vi "AprilTag Target Package Code 2.vi"() -> ()   [LabVIEW 2025]
uses:
  Camera Info.ctl
  <vilib>/vision/Shape Detection.llb/ShapeDetectionMatchOptions.ctl
  <vilib>/vision/Pattern Matching.llb/IMAQ Match Range Setting.ctl
  <vilib>/vision/Pattern Matching.llb/IMAQ Curve Parameters.ctl
  State Machine/AprialTag Main Cluster.ctl
  State Machine/AprialTag States.ctl
  <vilib>/vision/Image Controls.llb/IMAQ Image.ctl
  Steam Type.ctl
  Camera Set Up/Event/Event Setup Types.ctl
  <vilib>/Utility/config.llb/Read Key (String).vi
  <vilib>/Utility/config.llb/Write Key (String).vi
  <vilib>/Utility/config.llb/NI_LVConfig.lvlib
  <vilib>/vision/NI_Vision_Development_Module.lvlib
  <vilib>/ptbypt/NI_PtbyPt.lvlib
panel:
  in  "Main":enum32{"Page 1", "Page 2"}(tab)
  out "Target Pitch":dbl[](array[numeric]) caption="Tag Pitch (deg)" format="%.1f"
  out "Target Yaw":dbl[](array[numeric]) caption="Tag Yaw (deg)" format="%.1f"
  out "Tag ID":i32[](array[numeric]) caption="Tag Number"
  out "Image":T1(plugin-control)
  in  "Camera Name":string="cam0"
  in  "Settings":bool
  in  "Save":bool
  in  "Tools":bool
  out "FPS":dbl format="%#.0f"
  out "Distance":dbl[](array[numeric]) caption="Tag Distance (in)" format="%.1f"
  out "Angle":dbl[](array[numeric]) caption="Center Angle (deg)" format="%.1f"
  out "Height":u32=360
  out "Width":u32=640
  out "Waveform Chart":dbl[](graph)
  out "Treshold":T1(plugin-control)
  in  "Curve Parameters":T2={"Extraction Mode"=0, "Edge Threshold"=100, "Edge Filter Size"=1, "Min Length"=10, "Row Search Step Size"=75, "Col Search Step Size"=75, "Max Endpoint Gap"=10, "Closed"=TRUE, "Subpixel"=FALSE} {"Max Endpoint Gap" min=0; "Col Search Step Size" min=1 max=255 step=1; "Row Search Step Size" min=1 max=255 step=1; "Min Length" min=0; "Edge Filter Size" items=["Fine", "Normal", "Controur Tracing"]; "Edge Threshold" min=1 max=65535 step=1; "Extraction Mode" items=["Normal", "Uniform Regions"]}
  in  "Minimum match score":dbl=100.0
  in  "Home":bool
  in  "Robot Calibration Cluster":T3={"Camera Height on robot (in)"=9.5, "Camera Angle on the robot (deg)"=2.5, "Camera FOV Vert View Angle (deg)"=26.5, "Camera FOV Hor View Angle (deg)"=68.5, "Camera Focal Length (mm)"=10.0, "Target size (in)"=6.5} {"Camera FOV Hor View Angle (deg)" format="%#_13g"; "Camera Focal Length (mm)" format="%#_13g"; "Target size (in)" format="%#_13g"; "Camera FOV Vert View Angle (deg)" format="%#_13g"; "Camera Angle on the robot (deg)" format="%#_13g"; "Camera Height on robot (in)" format="%#_13g"}
  in  "Max Rect Size (pix)":dbl=12000.0
  in  "Min Rect Size (pix)":dbl=50.0
  in  "Match Options":T4={"Rotation"=TRUE, "Scale"=TRUE, "Occlusion"=FALSE, "Range Settings"=[{"Match Constraints"=0, "Min"=-25.0, "Max"=25.0}, {"Match Constraints"=1, "Min"=25.0, "Max"=200.0}]} {"Range Settings"."Match Constraints" items=["Rotation Angle (degrees)", "Scale Factor (%)", "Occlusion (%)"]}
  in  "Range":cluster{"Lower value":sgl, "Upper value":sgl}={"Lower value"=128.0, "Upper value"=255.0} {"Upper value" format="%.2f"; "Lower value" format="%.2f"}
  # "Edit the camera name to the camera that you are going to use for this target package"
  # "Range"
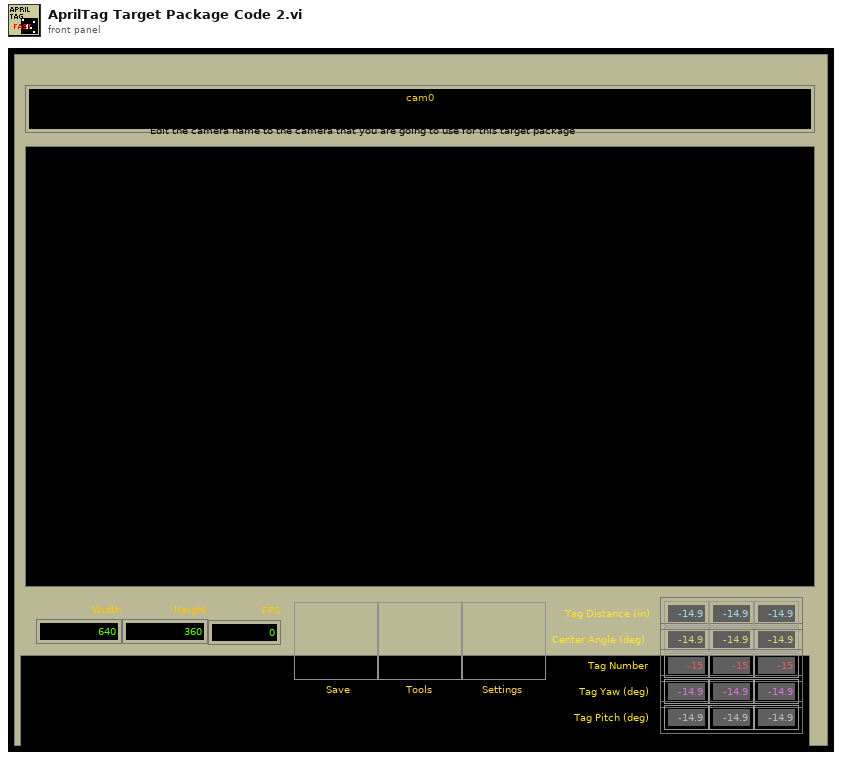
[diagram p1: front panel]
types:
  T1 = typedef "IMAQ Image.ctl" = refnum<image>
  T2 = typedef "IMAQ Curve Parameters.ctl" = cluster{"Extraction Mode":u32, "Edge Threshold":i32, "Edge Filter Size":u32, "Min Length":i32, "Row Search Step Size":i32, "Col Search Step Size":i32, "Max Endpoint Gap":i32, "Closed":bool, "Subpixel":bool}
  T3 = typedef "Camera Info.ctl" = cluster{"Camera Height on robot (in)":dbl, "Camera Angle on the robot (deg)":dbl, "Camera FOV Vert View Angle (deg)":dbl, "Camera FOV Hor View Angle (deg)":dbl, "Camera Focal Length (mm)":dbl, "Target size (in)":dbl}
  T4 = typedef "ShapeDetectionMatchOptions.ctl" = cluster{"Rotation":bool, "Scale":bool, "Occlusion":bool, "Range Settings":T5[]}
  T5 = typedef "IMAQ Match Range Setting.ctl" = cluster{"Match Constraints":u32, "Min":dbl, "Max":dbl}
  T6 = typedef "AprialTag States.ctl" = enum16{"Message Dispatcher", "INI", "Open", "Save", "Exit"}
  T7 = typedef "AprialTag Main Cluster.ctl" = cluster{"AprilTage FIFO":T6[], "Camera Name":string, "AprilTag path":path, "Control Ref's":refnum<vi>[], "Main Image":T1, "EDIT Settings":bool, "Calibration path":path, "Camera Number":dbl}
  T8 = cluster{"Min Width":dbl, "Max Width":dbl, "Min Height":dbl, "Max Height":dbl}
  T9 = typedef "Steam Type.ctl" = enum8{"Unknown", "Apriltag", "Fuel", "Other"}
  T10 = typedef "Event Setup Types.ctl" = enum16{"Default", "Camera Loop Started", "GreyScale", "Reset Team Number", "Save Data", "Exit"}
  T11 = typedef "Image Type" = u32
  T12 = cluster{"Corners":cluster{"X":sgl, "Y":sgl}[], "Angle":dbl, "Width":dbl, "Height":dbl, "Score":dbl}[]
  T13 = typedef "AprilTag Target Fields.ctl" = cluster{"diameter points":cluster{"first point":cluster{"x":dbl, "y":dbl}, "projected point":cluster{"x":dbl, "y":dbl}}, "normalized center":cluster{"x":dbl, "y":dbl}, "Overall Score":dbl, "Distance (ft)":dbl, "Offset Angle":dbl, "Tag corner points":cluster{"X":dbl, "Y":dbl}[], "Tag Center":cluster{"X":dbl, "Y":dbl}, "Tag Yaw":dbl, "Tag Pitch":dbl, "Target Roll (deg)":dbl, "AprilTag Number":i32, "homography matrix":dbl[]}
  T14 = typedef "NI_LVConfig.lvlib/Config Data RefNum.ctl" = refnum<k1>
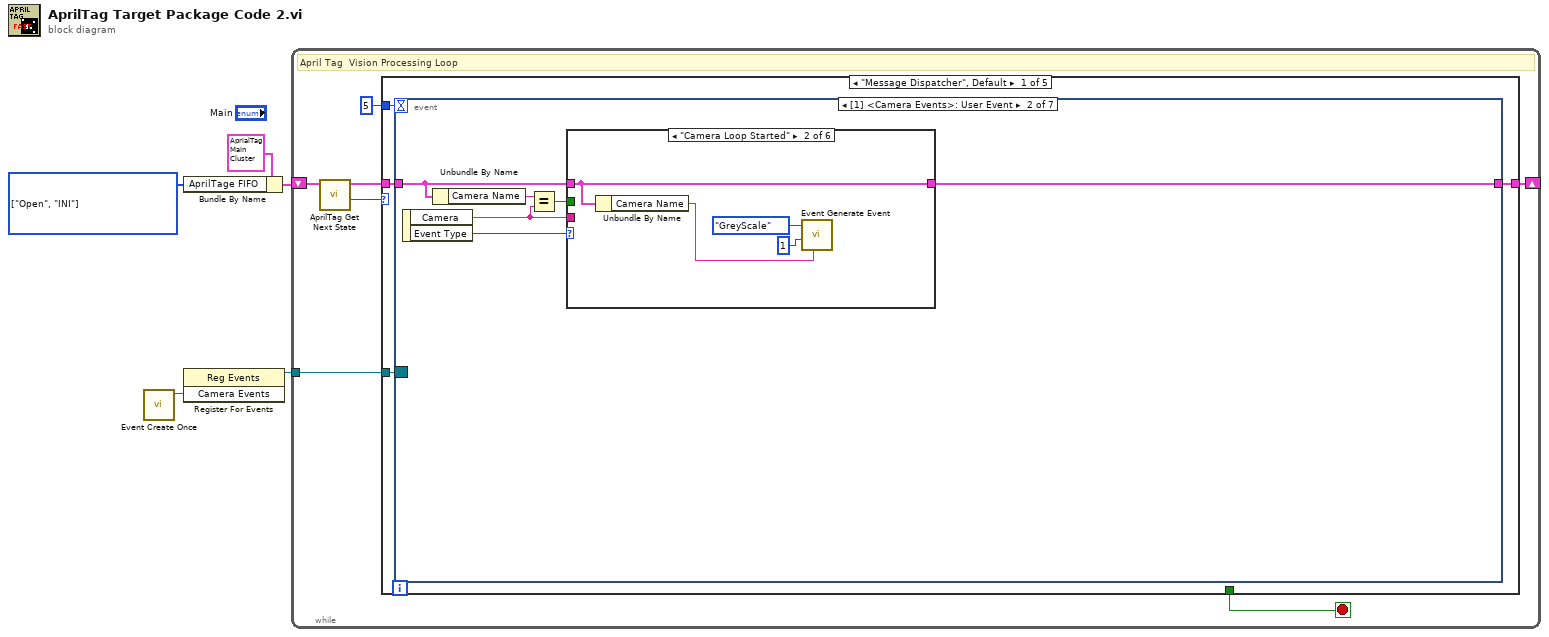
[diagram p0: block diagram]
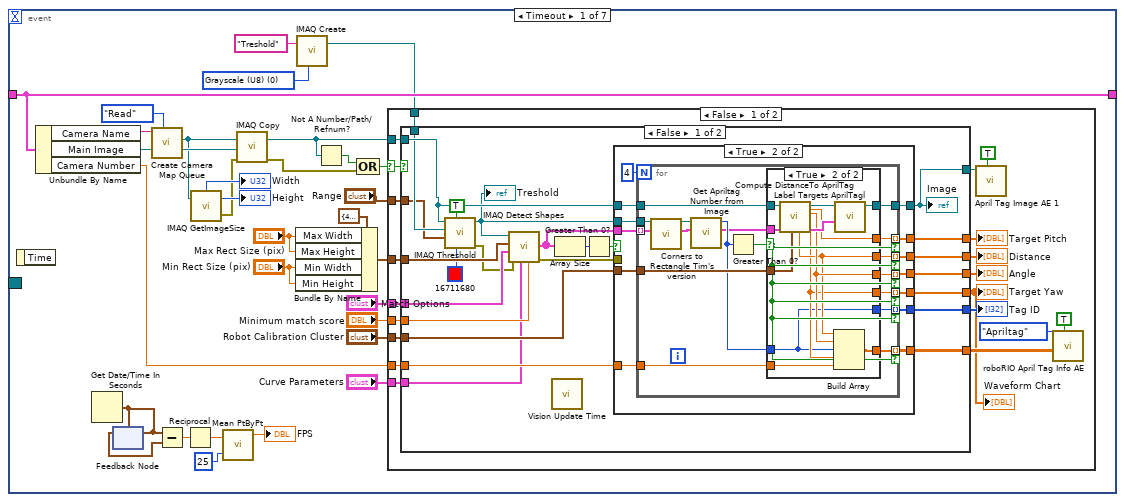
[diagram p2: hidden frame]
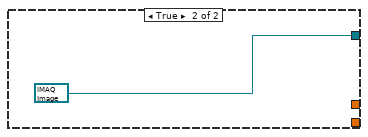
[diagram p5: hidden frame]
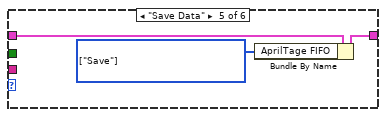
[diagram p10: hidden frame]
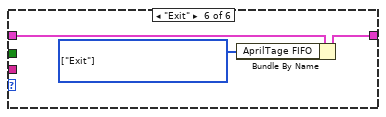
[diagram p11: hidden frame]
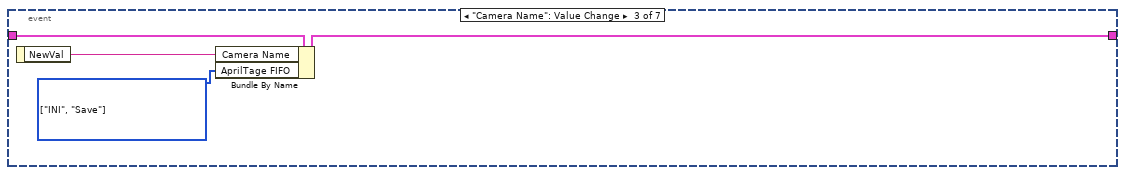
[diagram p12: hidden frame]
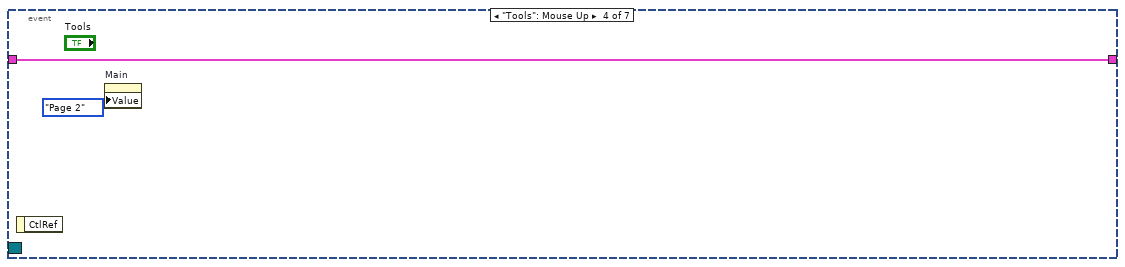
[diagram p13: hidden frame]
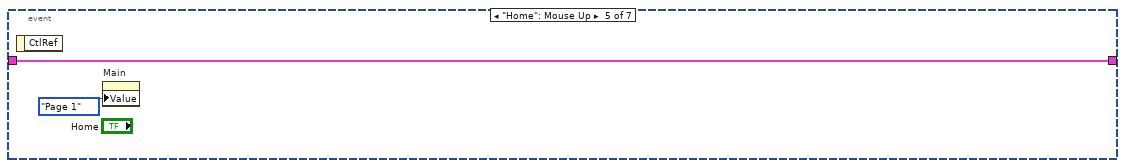
[diagram p14: hidden frame]
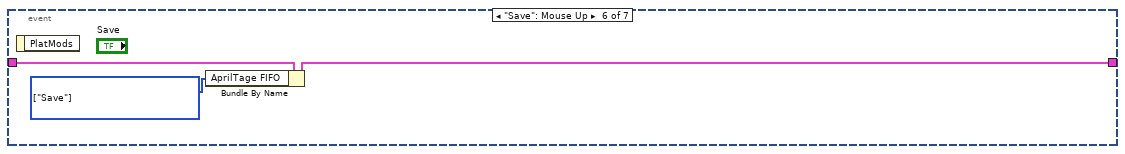
[diagram p15: hidden frame]
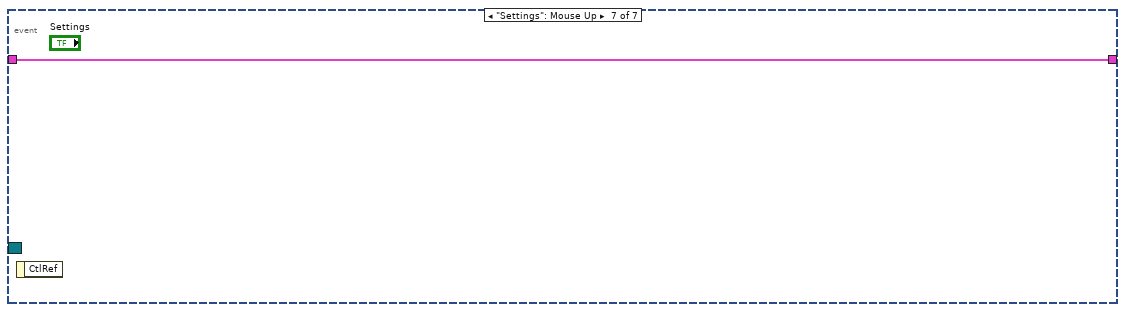
[diagram p16: hidden frame]
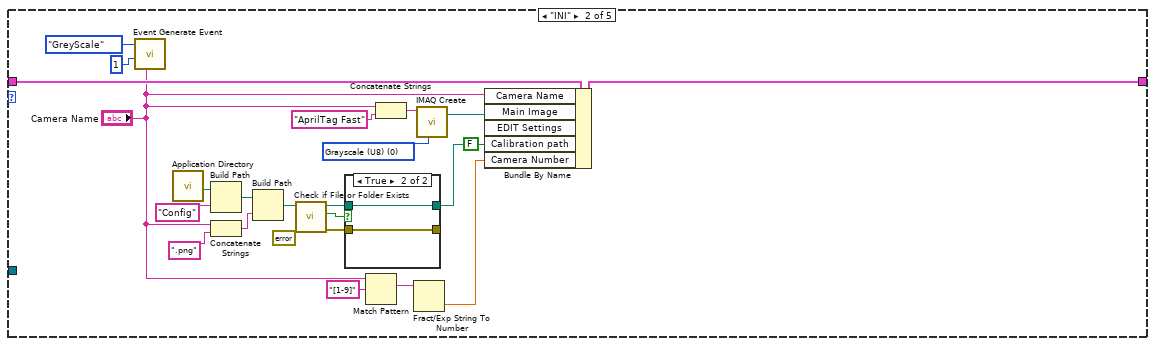
[diagram p17: hidden frame]
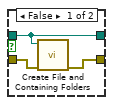
[diagram p18: hidden frame]
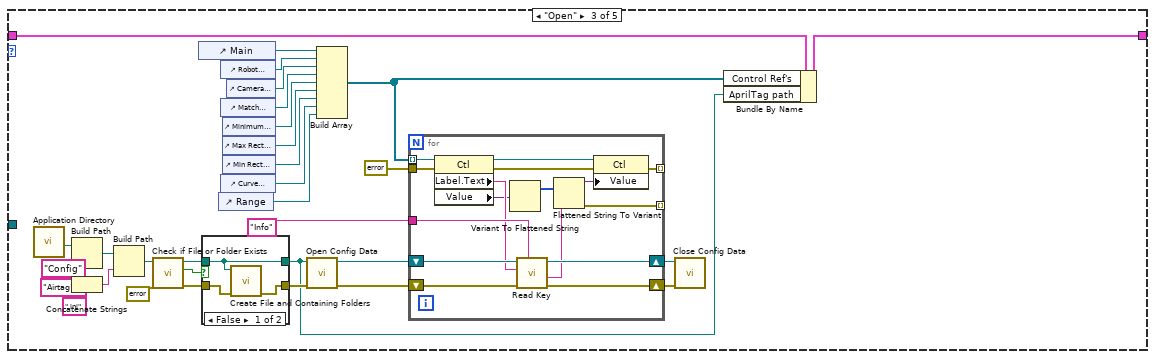
[diagram p19: hidden frame]
diagram:
  w1 = T6[] [enum."Open", enum."INI"] items=["Message Dispatcher", "INI", "Open", "Save", "Exit"] ("AprilTage FIFO")
  n1 = call "Event Create Once.vi"() -> ("Camera Events"=w5:refnum<user-event>)  [unwired: 10 in, 1 out]
  n2 = Bundle By Name(cluster=T7 {"AprilTage FIFO"=[], "Camera Name"="", "AprilTag path"=path "", "Control Ref's"=[], "Main Image"=refnum, "EDIT Settings"=FALSE, "Calibration path"=path "", "Camera Number"=0.0} ("AprilTag Main Cluster out"), "AprilTage FIFO"=w1) -> (w2:T7)
  n3 = register-events(w5) -> (reference out=w4:refnum<event-registration>)  [unwired: 2 in, 1 out]
  n4 = while {
    tunnel: w4 -> [w12]
    shift-right: [w8] -> _
    shift-left: w2 -> [w7]
    stop <- w11 stop-if-true
    # "April Tag  Vision Processing Loop"
    n5 = call "AprilTag Get Next State.vi"("AprilTag Main Cluster in"=w7) -> ("Next State"=w9:T6, "AprilTag Main Cluster out"=w10:T7)  [unwired: 9 in]
    n6 = case shown="\"Message Dispatcher\", Default" w9 {
      tunnel: w12 -> [w16 _ _ _ _]
      tunnel: [_ _ _ _ TRUE] -> w11
      tunnel: w10 -> [w14 w191 w214 w252 w268]
      tunnel: [w15 w190 w212 w252 w268] -> w8
      tunnel: 5 ("Timeout") -> [w13 _ _ _ _]
      frame "Message Dispatcher", Default {
        n7 = event shown="[1] <Camera Events>: User Event" {
          selector: w16 -> [_ _ _ _ _ _ _]
          dyn-events: _ -> [_ _ _ _ _ _ _]
          timeout: w13 -> [_ _ _ _ _ _ _]
          tunnel: w14 -> [w47 w140 w159 w160 w162 w166 w167]
          tunnel: [w47 w142 w158 w160 w162 w165 w167] -> w15
          event Timeout {
            w20 = T11 0 items=["Grayscale (U8)", "Grayscale (I16)", "Grayscale (SGL)", "Complex (CSG)", "RGB (U32)", "HSL (U32)", "RGB (U64)", "Grayscale (U16)"] ("Image Type")
            n8 = event-data() -> ()  [unwired: 1 in, 1 out]
            n9 = Unbundle By Name(w47) -> ("Camera Name"=w45:string, "Main Image"=w27:T1, "Camera Number"=w44:dbl)
            n10 = Get Date/Time In Seconds() -> (seconds since 1Jan1904=w33:timestamp)
            n11 = feedback-in #1(w33) -> ()
            n12 = feedback #1(w33) -> (w34:timestamp)
            n13 = call "Create Camera Map Queue.vi"("Action"=enum16{"Read", "Write"}."Read", "Camera"=w45) -> ("Image out"=w24:T1)  [unwired: 8 in, 1 out]
            n14 = Subtract(x=w33, y=w34) -> (x-y=w32:dbl)
            n15 = Reciprocal(x=w32) -> (1/x=w31:dbl)
            n16 = call "IMAQ GetImageSize"("Image"=w24) -> ("Y Resolution"=→"Height":i32, "X Resolution"=→"Width":i32, "error out"=w21:errorcluster)  [unwired: 3 in]
            n17 = call <vilib>:"Mean PtByPt.vi"("x"=w31, "sample length"=25) -> ("mean"=→"FPS":dbl)  [unwired: 2 in, 1 out]
            n18 = call "IMAQ Copy"("error in (no error)"=w21, "Image Dst"=w27, "Image Src"=w24) -> ("error out"=w25:errorcluster, "Image Dst Out"=w26:T1)  [unwired: 3 in]
            n19 = Bundle By Name(cluster=T8 {"Min Width"=40.0, "Max Width"=100.0, "Min Height"=40.0, "Max Height"=200.0} ("Rectangle Descriptor"), "Max Width"="Max Rect Size (pix)", "Max Height"="Max Rect Size (pix)", "Min Width"="Min Rect Size (pix)", "Min Height"="Min Rect Size (pix)") -> (w43:T8)
            n20 = call "IMAQ Create"("Image Name"="Treshold", "Image Type"=w20) -> ("New Image"=w18:T1)  [unwired: 2 in, 2 out]
            n21 = Not A Number/Path/Refnum?(number/path/refnum=w26) -> (NaN/Path/Refnum?=w36:bool)
            n22 = Compound Arithmetic op=OR(w36, w25) -> (w35:bool)
            n23 = case shown="False" w35 {
              selector: w35 -> [w51 _]
              tunnel: "Robot Calibration Cluster" -> [w66 _]
              tunnel: w26 -> [w61 _]
              tunnel: w44 -> [w60 _]
              tunnel: w43 -> [w58 _]
              tunnel: "Match Options" -> [w57 _]
              tunnel: "Minimum match score" -> [w56 _]
              tunnel: "Curve Parameters" -> [w52 _]
              tunnel: w18 -> [w50 _]
              tunnel: "Range" -> [w49 _]
              frame False {
                n24 = case shown="False" w51 {
                  tunnel: w66 -> [w91 _]
                  tunnel: [w89 _] -> w67
                  tunnel: [w88 _] -> w65
                  tunnel: [w87 _] -> w48
                  tunnel: [w86 _] -> w64
                  tunnel: [w85 _] -> w63
                  tunnel: [w84 _] -> w62
                  tunnel: w61 -> [w74 _]
                  tunnel: w60 -> [w83 _]
                  tunnel: [w82 T1 refnum ("Image out")] -> w59
                  tunnel: w58 -> [w81 _]
                  tunnel: w57 -> [w78 _]
                  tunnel: w56 -> [w77 _]
                  tunnel: w52 -> [w75 _]
                  tunnel: w50 -> [w72 _]
                  tunnel: w49 -> [w71 _]
                  frame False {
                    n25 = call "IMAQ Threshold"("Replace Value"=u32 16711680, "Keep/Replace Value (Replace)"=TRUE, "Range"=w71, "Image Dst"=w72, "Image Src"=w74) -> ("error out"=w69:errorcluster, "Image Dst Out"=w68:T1)  [unwired: 5 in]
                    "Treshold" <- w68
                    n26 = call-poly "IMAQ Detect Shapes"("Minimum match score"=w77, "Curve Parameters"=w75, "error in (no error)"=w69, "Match Options"=w78, "Rectangle Descriptor"=w81, "Image"=w68) -> ("error out"=w79:errorcluster, "Rectangles"=w80:T12)  [unwired: 3 in, 1 out]
                    n27 = call "Vision Update Time.vi"() -> ()  [unwired: 12 in]
                    n28 = Array Size(array=w80) -> (size(s)=w76:i32)
                    n29 = Greater Than 0?(x=w76) -> (x > 0?=w90:bool)
                    n30 = case shown="True" w90 {
                      tunnel: w74 -> [w92 w94]
                      tunnel: w80 -> [_ w105]
                      tunnel: [w92 w96] -> w82
                      tunnel: w91 -> [_ w104]
                      tunnel: [_ w103] -> w89
                      tunnel: [_ w102] -> w88
                      tunnel: [_ w101] -> w87
                      tunnel: [_ w100] -> w86
                      tunnel: [_ w99] -> w85
                      tunnel: [_ w98] -> w84
                      tunnel: w83 -> [_ w97]
                      tunnel: w79 -> [_ _]
                      tunnel: w68 -> [_ w95]
                      frame False {
                      }
                      frame True {
                        n31 = for {
                          N: 4 -> [_]
                          tunnel: w105 -> [w120] mode=indexing
                          tunnel: w94 -> [w112]
                          tunnel: [w121] -> w96
                          tunnel: [w106] -> w100 mode=indexing if=w107
                          tunnel: [w117] -> w98 mode=indexing if=w107
                          tunnel: [w119] -> w99 mode=indexing if=w107
                          tunnel: w104 -> [w118]
                          tunnel: [w116] -> w101 mode=indexing if=w107
                          tunnel: [w115] -> w103 mode=indexing if=w107
                          tunnel: [w114] -> w102 mode=indexing if=w107
                          tunnel: w97 -> [w113]
                          tunnel: w95 -> [w110]
                          n32 = call "Corners to Rectangle Tim's version.vi"("Rectangle Descriptor"=w120) -> ("tag info out"=w109:T13)  [unwired: 10 in]
                          n33 = call "Get Apriltag Number from Image.vi"("tag info"=w109, "Image"=w110) -> ("tag info out"=w108:T13, "AprilTag#"=w111:i32)  [unwired: 7 in, 1 out]
                          n34 = Greater Than 0?(x=w111) -> (x > 0?=w107:bool)
                          n35 = case shown="True" w107 {
                            tunnel: [w122 w135] -> w121
                            tunnel: w108 -> [_ w134]
                            tunnel: [_ w131] -> w119
                            tunnel: w118 -> [_ w130]
                            tunnel: [_ w129] -> w117
                            tunnel: [_ w128] -> w116
                            tunnel: [_ w127] -> w115
                            tunnel: [_ w126] -> w114
                            tunnel: w113 -> [_ w125]
                            tunnel: w112 -> [w122 w124]
                            tunnel: w111 -> [_ w123]
                            tunnel: [_ w123] -> w106
                            frame False {
                            }
                            frame True {
                              n36 = call "Compute DistanceTo AprilTag.vi"("Robot Calibration Cluster"=w130, "results"=w134, "Image Src"=w124) -> ("results out"=w133:T13, "Target Yaw (deg)"=w128:dbl, "Offset Angle"=w131:dbl, "Image Dst Out"=w132:T1, "Distance from target (in)"=w129:dbl, "Target Pitch (deg)"=w126:dbl)  [unwired: 3 in]
                              n37 = Build Array(w129, w131, w123, w128, w125) -> (w127:dbl[])
                              n38 = call "Label Targets AprilTagl.vi"("results"=w133, "Image in"=w132) -> ("Image out"=w135:T1)  [unwired: 9 in]
                            }
                          }
                        }
                      }
                    }
                    "Image" <- w82
                  }
                  frame True {
                  }
                }
                "Distance" <- w62
                "Angle" <- w63
                "Tag ID" <- w64
                "Target Yaw" <- w48
                "Target Pitch" <- w65
                "Waveform Chart" <- w48
                n39 = call "April Tag Image AE 1.vi"("Update"=TRUE, "Apriltag Image in"=w59) -> ()  [unwired: 9 in, 1 out]
                n40 = call "roboRIO April Tag Info AE.vi"("Update"=TRUE, "Info in"=w67, "Stream Type"=Steam_Type."Apriltag") -> ()  [unwired: 8 in, 1 out]
              }
              frame True {
              }
            }
          }
          event User Event {
            n41 = event-data() -> ("Camera"=w137:string, "Event Type"=w141:T10)  [unwired: 1 in]
            n42 = Unbundle By Name(w140) -> ("Camera Name"=w139:string)
            n43 = Equal?(x=w139, y=w137) -> (x = y?=w138:bool)
            n44 = case shown="\"Camera Loop Started\"" w141 {
              tunnel: w140 -> [w143 w145 w148 w149 w152 w155]
              tunnel: [w143 w145 w148 w149 w151 w154] -> w142
              tunnel: w138 -> [_ _ _ _ _ _]
              tunnel: w137 -> [_ _ _ _ _ _]
              frame "Default" {
              }
              frame "Camera Loop Started" {
                n45 = Unbundle By Name(w145) -> ("Camera Name"=w144:string)
                n46 = call "Event Generate Event.vi"("Camera Name"=w144, "Setpoint"=i64 1, "Event Type"=Event_Setup_Types."GreyScale") -> ()  [unwired: 9 in]
              }
              frame "GreyScale" {
              }
              frame "Reset Team Number" {
              }
              frame "Save Data" {
                w150 = T6[] [enum."Save"] items=["Message Dispatcher", "INI", "Open", "Save", "Exit"] ("AprilTage FIFO")
                n47 = Bundle By Name(cluster=w152, "AprilTage FIFO"=w150) -> (w151:T7)
              }
              frame "Exit" {
                w153 = T6[] [enum."Exit"] items=["Message Dispatcher", "INI", "Open", "Save", "Exit"] ("AprilTage FIFO")
                n48 = Bundle By Name(cluster=w155, "AprilTage FIFO"=w153) -> (w154:T7)
              }
            }
          }
          event "Camera Name": Value Change {
            w157 = T6[] [enum."INI", enum."Save"] items=["Message Dispatcher", "INI", "Open", "Save", "Exit"] ("AprilTage FIFO")
            n49 = event-data() -> ("NewVal"=w156:string)  [unwired: 1 in]
            n50 = Bundle By Name(cluster=w159, "Camera Name"=w156, "AprilTage FIFO"=w157) -> (w158:T7)
          }
          event "Tools": Mouse Up {
            n51 = event-data() -> ()  [unwired: 1 in, 1 out]
            n52 = property on="Main" class="TabCtl (strict)"("Value"=enum32{"Page 1", "Page 2"}."Page 2" ("Main")) -> ()  [unwired: 2 in, 2 out]
          }
          event "Home": Mouse Up {
            n53 = event-data() -> ()  [unwired: 1 in, 1 out]
            n54 = property on="Main" class="TabCtl (strict)"("Value"=enum32{"Page 1", "Page 2"}."Page 1" ("Main")) -> ()  [unwired: 2 in, 2 out]
          }
          event "Save": Mouse Up {
            w164 = T6[] [enum."Save"] items=["Message Dispatcher", "INI", "Open", "Save", "Exit"] ("AprilTage FIFO")
            n55 = event-data() -> ()  [unwired: 1 in, 1 out]
            n56 = Bundle By Name(cluster=w166, "AprilTage FIFO"=w164) -> (w165:T7)
          }
          event "Settings": Mouse Up {
            n57 = event-data() -> ()  [unwired: 1 in, 1 out]
          }
        }
      }
      frame "INI" {
        w189 = T11 0 items=["Grayscale (U8)", "Grayscale (I16)", "Grayscale (SGL)", "Complex (CSG)", "RGB (U32)", "HSL (U32)", "RGB (U64)", "Grayscale (U16)"] ("Image Type")
        n58 = call "Event Generate Event.vi"("Camera Name"="Camera Name", "Setpoint"=i64 1, "Event Type"=Event_Setup_Types."GreyScale") -> ()  [unwired: 9 in]
        n59 = call <vilib>:"Application Directory.vi"() -> ("Application Directory"=w182:path)
        n60 = Build Path(base path=w182, name or relative path="Config") -> (appended path=w180:path)
        n61 = Concatenate Strings("Camera Name", ".png" ("name or relative path")) -> (w184:string)
        n62 = Build Path(base path=w180, name or relative path=w184) -> (appended path=w179:path)
        n63 = call <vilib>:"Check if File or Folder Exists.vi"("error in (no error)"=errorcluster {"status"=FALSE, "code"=0, "source"=""}, "path"=w179) -> ("error out"=w176:errorcluster, "file or folder exists?"=w177:bool, "dup path"=w178:path)  [unwired: 7 in]
        n64 = case shown="True" w177 {
          tunnel: [w194 w195] -> _
          tunnel: w178 -> [w193 w196]
          tunnel: [w193 w196] -> w174
          tunnel: w176 -> [w192 w195]
          frame False {
            n65 = call <vilib>:"Create File and Containing Folders.vi"("error in (no error)"=w192, "file path"=w193) -> ("error out"=w194:errorcluster)  [unwired: 8 in, 1 out]
          }
          frame True {
          }
        }
        n66 = Match Pattern(string="Camera Name", regular expression="[1-9]") -> (match substring=w172:string)  [unwired: 1 in, 3 out]
        n67 = Concatenate Strings("Camera Name", "AprilTag Fast" ("string")) -> (w188:string)
        n68 = Fract/Exp String To Number(string=w172) -> (number=w171:dbl)  [unwired: 3 in, 1 out]
        n69 = call "IMAQ Create"("Image Name"=w188, "Image Type"=w189) -> ("New Image"=w186:T1)  [unwired: 2 in, 2 out]
        n70 = Bundle By Name(cluster=w191, "Camera Name"="Camera Name", "Main Image"=w186, "EDIT Settings"=FALSE, "Calibration path"=w174, "Camera Number"=w171) -> (w190:T7)
      }
      frame "Open" {
        n71 = call <vilib>:"Application Directory.vi"() -> ("Application Directory"=w217:path)
        n72 = Build Path(base path=w217, name or relative path="Config") -> (appended path=w215:path)
        n73 = Concatenate Strings("Airtag1" ("string"), ".ini" ("name or relative path")) -> (w227:string)
        n74 = Build Path(base path=w215, name or relative path=w227) -> (appended path=w208:path)
        n75 = call <vilib>:"Check if File or Folder Exists.vi"("error in (no error)"=errorcluster {"status"=FALSE, "code"=0, "source"=""}, "path"=w208) -> ("error out"=w204:errorcluster, "file or folder exists?"=w206:bool, "dup path"=w207:path)  [unwired: 7 in]
        n76 = control-ref of="Main"() -> (w222:refnum<vi>)
        n77 = case shown="False" w206 {
          tunnel: [w230 w231] -> w218
          tunnel: w207 -> [w229 w232]
          tunnel: [w229 w232] -> w205
          tunnel: w204 -> [w228 w231]
          frame False {
            n78 = call <vilib>:"Create File and Containing Folders.vi"("error in (no error)"=w228, "file path"=w229) -> ("error out"=w230:errorcluster)  [unwired: 8 in, 1 out]
          }
          frame True {
          }
        }
        n79 = control-ref of="Range"() -> (w197:refnum<vi>)
        n80 = control-ref of="Robot Calibration Cluster"() -> (w221:refnum<vi>)
        n81 = control-ref of="Match Options"() -> (w202:refnum<vi>)
        n82 = control-ref of="Curve Parameters"() -> (w198:refnum<vi>)
        n83 = control-ref of="Minimum match score"() -> (w201:refnum<vi>)
        n84 = control-ref of="Max Rect Size (pix)"() -> (w200:refnum<vi>)
        n85 = control-ref of="Min Rect Size (pix)"() -> (w199:refnum<vi>)
        n86 = control-ref of="Camera Name"() -> (w213:refnum<vi>)
        n87 = call <vilib>:"Open Config Data.vi"("error in (no error)"=w218, "configuration file path"=w205) -> ("error out"=w223:errorcluster, "refnum"=w226:T14)  [unwired: 7 in, 1 out]
        n88 = Build Array(w222, w221, w213, w202, w201, w200, w199, w198, w197) -> (w211:refnum<vi>[])
        n89 = for {
          tunnel: "Info" ("Camera Name") -> [w245]
          tunnel: w211 -> [w243] mode=indexing
          shift-right: [w247] -> w225
          shift-left: w226 -> [w248]
          shift-right: [w246] -> w224
          shift-left: w223 -> [w244]
          tunnel: [w238] -> _ mode=indexing
          tunnel: errorcluster {"status"=FALSE, "code"=0, "source"=""} ("error out") -> [w237]
          tunnel: [w233] -> _ mode=indexing
          n90 = property class="Ctl"(reference=w243, error in=w237) -> (reference out=w241:refnum<vi>, error out=w239:errorcluster, "Label.Text"=w242:string, "Value"=w235:variant)
          n91 = Variant To Flattened String(Variant=w235) -> (1:w234:i16[])  [unwired: 1 out]
          n92 = call-poly <vilib>:"Read Key.vi"("section"=w245, "error in (no error)"=w244, "key"=w242, "refnum"=w248) -> ("error out"=w246:errorcluster, "value"=w240:string, "refnum out"=w247:T14)  [unwired: 4 in, 1 out]
          n93 = Flattened String To Variant(6:w240, 7:w234) -> (0:w233:errorcluster, 3:w236:variant)  [unwired: 1 in]
          n94 = property class="Ctl"(reference=w241, error in=w239, "Value"=w236) -> (error out=w238:errorcluster)  [unwired: 1 out]
        }
        n95 = call <vilib>:"Close Config Data.vi"("error in (no error)"=w224, "refnum"=w225) -> ()  [unwired: 8 in, 2 out]
        n96 = Bundle By Name(cluster=w214, "Control Ref's"=w211, "AprilTag path"=w205) -> (w212:T7)
      }
      frame "Save" {
        n97 = Unbundle By Name(w252) -> ("Control Ref's"=w250:refnum<vi>[], "AprilTag path"=w251:path)
        n98 = call <vilib>:"Open Config Data.vi"("configuration file path"=w251) -> ("error out"=w253:errorcluster, "refnum"=w256:T14)  [unwired: 8 in, 1 out]
        n99 = for {
          tunnel: "Info" ("Camera Name") -> [w262]
          shift-right: [w265] -> w255
          shift-left: w256 -> [w266]
          shift-right: [w264] -> w254
          shift-left: w253 -> [w263]
          tunnel: w250 -> [w257] mode=indexing
          n100 = property class="Ctl"(reference=w257, error in=w263) -> (error out=w259:errorcluster, "Label.Text"=w261:string, "Value"=w260:variant)  [unwired: 1 out]
          n101 = Variant To Flattened String(Variant=w260) -> (data string=w258:string)  [unwired: 1 out]
          n102 = call-poly <vilib>:"Write Key.vi"("section"=w262, "error in (no error)"=w259, "value"=w258, "key"=w261, "refnum"=w266) -> ("error out"=w264:errorcluster, "refnum out"=w265:T14)  [unwired: 4 in, 1 out]
        }
        n103 = call <vilib>:"Close Config Data.vi"("error in (no error)"=w254, "refnum"=w255) -> ()  [unwired: 8 in, 2 out]
      }
      frame "Exit" {
        n104 = Unbundle By Name(w268) -> ("Main Image"=w267:T1)
        n105 = call "IMAQ Dispose"("Image"=w267) -> ()  [unwired: 5 in, 1 out]
      }
    }
  }
